vi "TL forebrain SENSE.vi"(2 "error in":errorcluster, 3 "Stuck?":bool, 4 "Boat Status":T1) -> (0 "error out":errorcluster, 1 "GPS":cluster{"X pos":i32, "Y pos":i32, "Heading":dbl})   [LabVIEW 2014]
uses:
  boatStatus.ctl
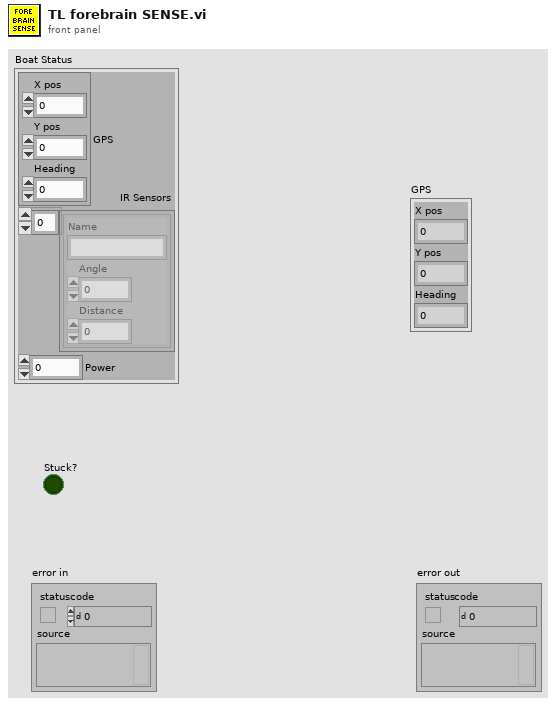
[diagram p1: front panel]
types:
  T1 = typedef "boatStatus.ctl" = cluster{"GPS":cluster{"X pos":i32, "Y pos":i32, "Heading":dbl}, "IR Sensors":cluster{"Name":string, "Angle":dbl, "Distance":dbl}[], "Power":dbl}
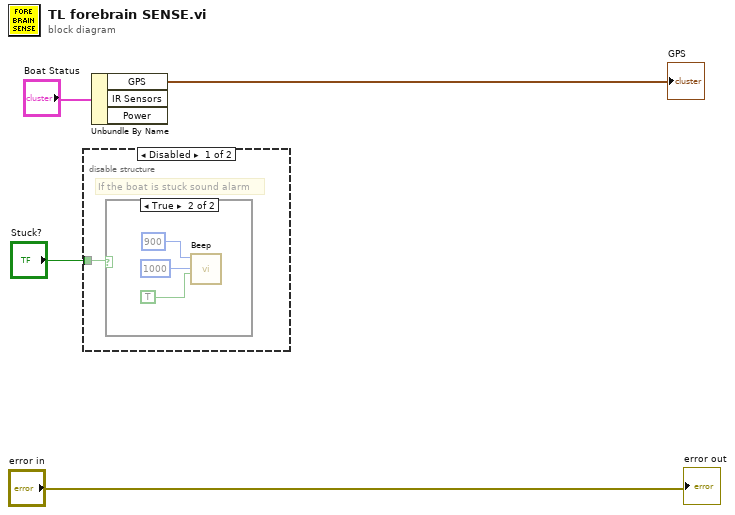
[diagram p0: block diagram]
diagram:
  n1 = disable-structure shown="Disabled" {
    disable-tunnel: "Stuck?" -> [w5 _]
    frame Disabled {
      # "If the boat is stuck sound alarm"
      n2 = case shown="True" w5 {
        frame False {
        }
        frame True {
          n3 = call <vilib>:"Beep.vi"("use system alert? (T)"=TRUE, "duration (msec)"=u32 1000, "frequency (Hz)"=u32 900) -> ()  [unwired: 9 in]
        }
      }
    }
    frame Enabled {
    }
  }
  n4 = Unbundle By Name("Boat Status") -> ("GPS"=→"GPS":cluster{"X pos":i32, "Y pos":i32, "Heading":dbl})  [unwired: 2 out]
  "error out" <- "error in"
